vi "Read Measurement (Transistor).vi"(0 "VISA resource name":refnum<visa-resource-name>, 5 "Quality Measurement Type (0: Rds(on))":i32(ring) items=["Rds(on)", "Vce(sat)"], 11 "error in (no error)":errorcluster) -> (4 "VISA resource name out":refnum<visa-resource-name>, 6 "Transistor Measurement":dbl, 15 "error out":errorcluster)   [LabVIEW 2015, in "Agilent 2000 3000 X-Series.lvlib"]
doc: "Returns a transistor measurement from the oscilloscope. Can read Rds(on) or Vce(sat)"
uses:
  <instrlib>/Agilent 2000 3000 X-Series/Agilent 2000 3000 X-Series.lvlib
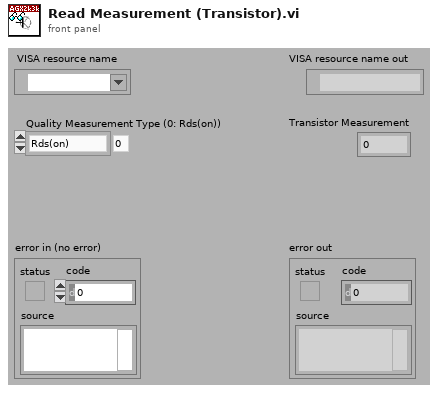
[diagram p1: front panel]
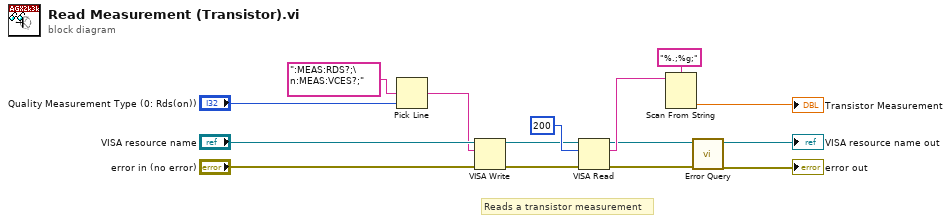
[diagram p0: block diagram]
diagram:
  # "Reads a transistor measurement"
  n1 = Pick Line(multi-line string=":MEAS:RDS?;\n:MEAS:VCES?;", line index="Quality Measurement Type (0: Rds(on))") -> (output string=w3:string)  [unwired: 1 out]
  n2 = VISA Write(VISA resource name="VISA resource name", write buffer=w3, error in (no error)="error in (no error)") -> (VISA resource name out=w9:refnum<visa-resource-name>, error out=w8:errorcluster)  [unwired: 1 out]
  n3 = VISA Read(VISA resource name=w9, byte count=u32 200, error in (no error)=w8) -> (VISA resource name out=w6:refnum<visa-resource-name>, read buffer=w10:string, error out=w7:errorcluster)  [unwired: 1 out]
  n4 = Scan From String(format string="%.;%g;", input string=w10) -> (output 1=→"Transistor Measurement":dbl)  [unwired: 2 in, 4 out]
  n5 = call <instrlib>:"Error Query.vi"("error in (no error)"=w7, "VISA resource name"=w6) -> ("error out"=→"error out":errorcluster, "VISA resource name out"=→"VISA resource name out":refnum<visa-resource-name>)  [unwired: 8 out]
